vi "Create.vi"(8 "error in (no error)":errorcluster, 11 "ICPCON ET-7017 in":refnum<class "ICPCON PM-3112.lvclass">) -> (0 "error out":errorcluster, 3 "ICPCON ET-7017 out":refnum<class "ICPCON PM-3112.lvclass">)   [LabVIEW 2021, in "ICPCON PM-3112.lvclass"]
uses:
  ICPCON PM-3112.lvclass
  D:/my_projects/projects/Algorithms/Labview/21/Master CR/Master CR.lvclass
  Data Model/ICPCON PM3114 Data Model/ICPCON PM3114 Data Model.lvclass
  D:/my_projects/projects/Algorithms/Labview/21/Modbus_v121c/Data Model/Device Data Model.lvclass
  Master CR.lvclass/Master CR.ctl
  TCP/TCP.lvclass
  ICPCON PM-3112.lvclass/ICPCON PM-3112.ctl
  Master CR.lvclass
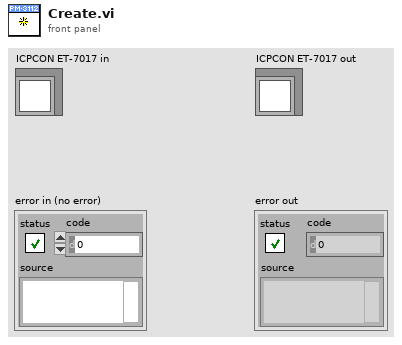
[diagram p1: front panel]
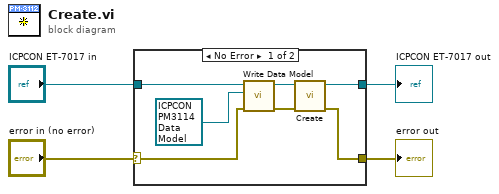
[diagram p0: block diagram]
diagram:
  n1 = case shown="No Error" "error in (no error)" {
    selector: "error in (no error)" -> [w5 w12]
    tunnel: [w9 w12] -> w1
    tunnel: [w10 w13] -> w2
    tunnel: "ICPCON ET-7017 in" -> [w11 w13]
    frame No Error {
      n2 = call "Write Data Model.vi"("error in (no error)"=w5, "Data Model"=refnum<class "ICPCON PM3114 Data Model.lvclass"> refnum ("Modbus API:Device Data Model"), "Master CR in"=w11) -> ("error out"=w8:errorcluster, "Master CR out"=w7:refnum<class "ICPCON PM-3112.lvclass">)  [unwired: 7 in]
      n3 = call-parent "Create.vi"("error in (no error)"=w8, "TCP in"=w7) -> ("error out"=w9:errorcluster, "TCP out"=w10:refnum<class "ICPCON PM-3112.lvclass">)  [unwired: 8 in]
    }
    frame Error {
    }
  }
  "error out" <- w1
  "ICPCON ET-7017 out" <- w2
